vi "ELOG_Channels_Set.vi"(8 "error in (no error)":errorcluster, 10 "Channel Name List":string[](array[string]), 11 "OXY_SCPI Reseource In":refnum<visa-resource-name>) -> (0 "error out":errorcluster, 1 "communication_data":T1, 3 "OXY_SCPI Reseource IOut":refnum<visa-resource-name>)   [LabVIEW 2018, in "OXYGEN.lvlib"]
doc: "Defines the ordered list of requested channels."
uses:
  OXYGEN.lvlib
  TypeDefs/Cluster_RawCommData.ctl
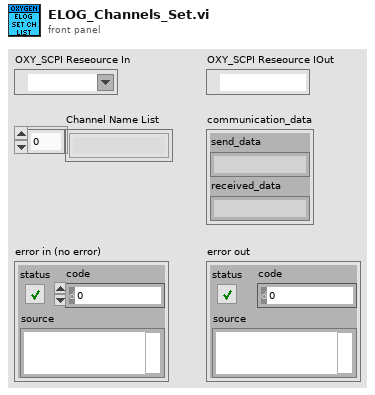
[diagram p1: front panel]
types:
  T1 = typedef "OXYGEN.lvlib/Cluster_RawCommData.ctl" = cluster{"send_data":string, "received_data":string}
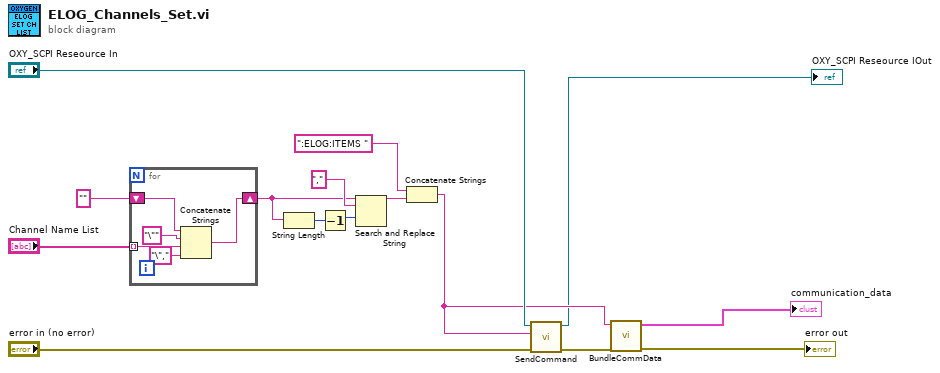
[diagram p0: block diagram]
diagram:
  n1 = for {
    tunnel: "Channel Name List" -> [w20] mode=indexing
    shift-right: [w16] -> w5
    shift-left: "" -> [w19]
    n2 = Concatenate Strings(w19, "\"" ("string"), w20, "\"," ("string")) -> (w16:string)
  }
  n3 = String Length(string=w5) -> (length=w6:i32)
  n4 = Decrement(x=w6) -> (x-1=w8:i32)
  n5 = Search and Replace String(input string=w5, search string=",", offset=w8) -> (result string=w4:string)  [unwired: 5 in, 3 out]
  n6 = Concatenate Strings(":ELOG:ITEMS " ("string"), w4) -> (w2:string)
  n7 = call "SendCommand.vi"("error in (no error)"="error in (no error)", "String to Send"=w2, "OXY_SCPI Reseource In"="OXY_SCPI Reseource In") -> ("error out"=w12:errorcluster, "OXY_SCPI Reseource Out"=→"OXY_SCPI Reseource IOut":refnum<visa-resource-name>)  [unwired: 7 in]
  n8 = call "BundleCommData.vi"("error in (no error)"=w12, "send_data"=w2) -> ("error out"=→"error out":errorcluster, "communication_data"=→"communication_data":T1)  [unwired: 8 in]
